vi "TestModuleSync.vi"() -> ()   [LabVIEW 2018, in "ModuleAdmin.lvlib" / "ModuleAdmin.lvclass"]
uses:
  ModuleAdmin.lvclass
panel:
  in  "ModuleName":string="Module"
  in  "ModuleID":i32=-1
  out "error out":errorcluster
  in  "error in (no error)":errorcluster
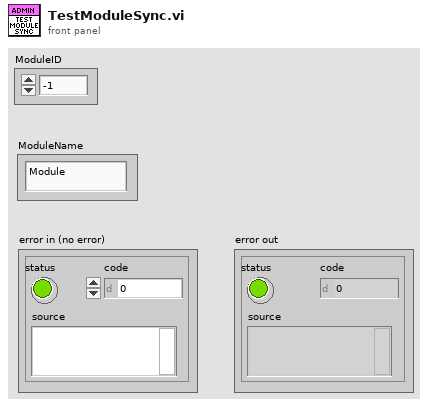
[diagram p1: front panel]
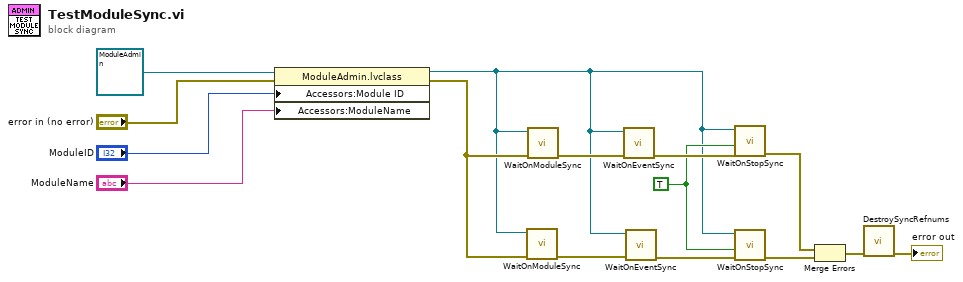
[diagram p0: block diagram]
diagram:
  w13 = TRUE ("WaitForModuleToStop?")
  n1 = property class="ModuleAdmin.lvclass"(reference=refnum<class "ModuleAdmin.lvclass"> refnum ("NistModuleAdmin.lvlib:NistModuleAdmin.lvclass"), error in="error in (no error)", "Accessors:Module ID"="ModuleID", "Accessors:ModuleName"="ModuleName") -> (reference out=w2:refnum<class "ModuleAdmin.lvclass">, error out=w3:errorcluster)
  n2 = call "WaitOnModuleSync.vi"("error in (no error)"=w3, "ModuleAdmin"=w2) -> ("error out"=w9:errorcluster)  [unwired: 8 in, 1 out]
  n3 = call "WaitOnModuleSync.vi"("error in (no error)"=w3, "ModuleAdmin"=w2) -> ("error out"=w15:errorcluster)  [unwired: 8 in, 1 out]
  n4 = call "WaitOnEventSync.vi"("error in (no error)"=w15, "ModuleAdmin"=w2) -> ("error out"=w14:errorcluster)  [unwired: 8 in, 1 out]
  n5 = call "WaitOnEventSync.vi"("error in (no error)"=w9, "ModuleAdmin"=w2) -> ("error out"=w8:errorcluster)  [unwired: 8 in, 1 out]
  n6 = call "WaitOnStopSync.vi"("error in (no error)"=w14, "WaitForModuleToStop?"=w13, "ModuleAdmin"=w2) -> ("error out"=w11:errorcluster)  [unwired: 7 in, 1 out]
  n7 = call "WaitOnStopSync.vi"("error in (no error)"=w8, "WaitForModuleToStop?"=w13, "ModuleAdmin"=w2) -> ("error out"=w10:errorcluster)  [unwired: 7 in, 1 out]
  n8 = Merge Errors(w11, w10) -> (w12:errorcluster)
  n9 = call "DestroySyncRefnums.vi"("error in (no error)"=w12) -> ("error out"=→"error out":errorcluster)  [unwired: 10 in]
